vi "WPI_AccumulatorReset.vi"(8 "error in (no error)":errorcluster, 11 "AIDeviceRef":T1={"DevStatus"={"status"=FALSE, "code"=0, "source"=""}, "Analog Channel"=enum."Invalid"}) -> (0 "error out":errorcluster, 3 "AIDeviceRef":T1={"DevStatus"={"status"=FALSE, "code"=0, "source"=""}, "Analog Channel"=enum."Invalid"})   [LabVIEW 2017]
doc: "Resets the accumulator on the FPGA on the roboRIO device to the initial value you set with the SetConfiguration VI. By default, the initial value is 0.\n\nThis software is licensed. Open the labview\\readme\\WPI Robotics Library Open Source License.txt file for more information."
uses:
  <vilib>/Rock Robotics/WPI/AnalogChannel/WPI_AnalogChannelDevRef.ctl
  <vilib>/Rock Robotics/SystemInterfaces/AI/FPGA_AIChannel.ctl
  <vilib>/Rock Robotics/SystemInterfaces/System/FPGA_SystemGet.vi
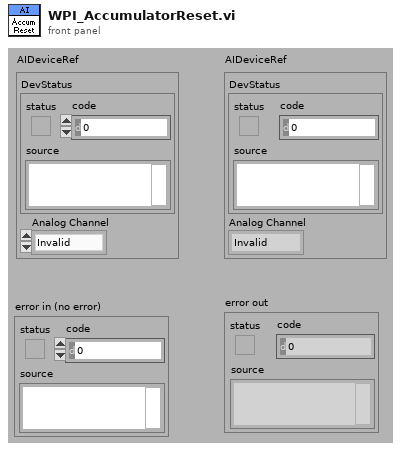
[diagram p1: front panel]
types:
  T1 = typedef "WPI_AnalogChannelDevRef.ctl" = cluster{"DevStatus":errorcluster, "Analog Channel":T2}
  T2 = typedef "FPGA_AIChannel.ctl" = enum8{"AI 0", "AI 1", "AI 2", "AI 3", "AI MXP 0", "AI MXP 1", "AI MXP 2", "AI MXP 3", "Invalid"}
  T3 = typedef "FPGA_AIDevRef.ctl" = cluster{"DevStatus":errorcluster}
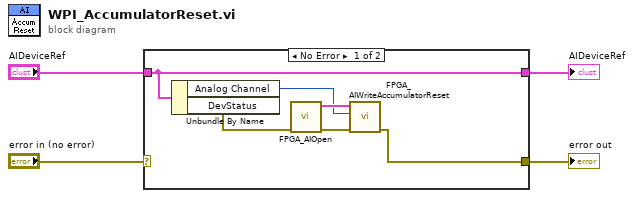
[diagram p0: block diagram]
diagram:
  n1 = case shown="No Error" "error in (no error)" {
    selector: "error in (no error)" -> [_ w11]
    tunnel: [w10 w12] -> w4
    tunnel: "AIDeviceRef" -> [w10 w12]
    tunnel: [w7 w11] -> w1
    frame No Error {
      n2 = Unbundle By Name(w10) -> ("Analog Channel"=w6:T2, "DevStatus"=w9:errorcluster)
      n3 = call <vilib>:"FPGA_AIOpen.vi"("error in (no error)"=w9) -> ("error out"=w5:errorcluster, "AI Reference out"=w8:T3)  [unwired: 2 in, 7 out]
      n4 = call <vilib>:"FPGA_AIWriteAccumulatorReset.vi"("error in (no error)"=w5, "Channel"=w6, "AI Reference in"=w8) -> ("error out"=w7:errorcluster)  [unwired: 8 out]
    }
    frame Error {
    }
  }
  "AIDeviceRef" <- w4
  "error out" <- w1
